vi "WPI_SonarSRF08_I2C_GetSetRefNum.vi"(8 "error in (no error)":errorcluster, 9 "menu":T1, 10 "refnum name":string, 11 "SonarSRF08_I2C_DevRef":T2={"I2CDevRef"={"DevStatus"={"status"=FALSE, "code"=0, "source"=""}, "Device Address"=0, "Handle"=0, "I2C Bus"=enum."Invalid"}} {"I2CDevRef"."Device Address" format="%.0x"}) -> (0 "error out":errorcluster, 2 "names":string[](array[string]), 3 "SonarSRF08_I2C_DevRef":T2={"I2CDevRef"={"DevStatus"={"status"=FALSE, "code"=0, "source"=""}, "Device Address"=0, "Handle"=0, "I2C Bus"=enum."Invalid"}} {"I2CDevRef"."Device Address" format="%.0x"})   [LabVIEW 2017]
doc: "Sets a reference into a registry, gets a reference from a registry, or deletes a reference from a registry. The reference is accessed by name, and can be given any unique name.\n\nThis software is licensed. Open the labview\\readme\\WPI Robotics Library Open Source License.txt file for more information."
uses:
  <vilib>/Rock Robotics/WPI/Ultrasonic/WPI_SonarSRF08_I2C_DeviceRef.ctl
  <vilib>/Rock Robotics/WPI/I2C/WPI_I2CDevRef.ctl
  <vilib>/Rock Robotics/SystemInterfaces/i2clib/i2c_bus.ctl
  <vilib>/Rock Robotics/WPI/Utilities/Refnum Registry Operation.ctl
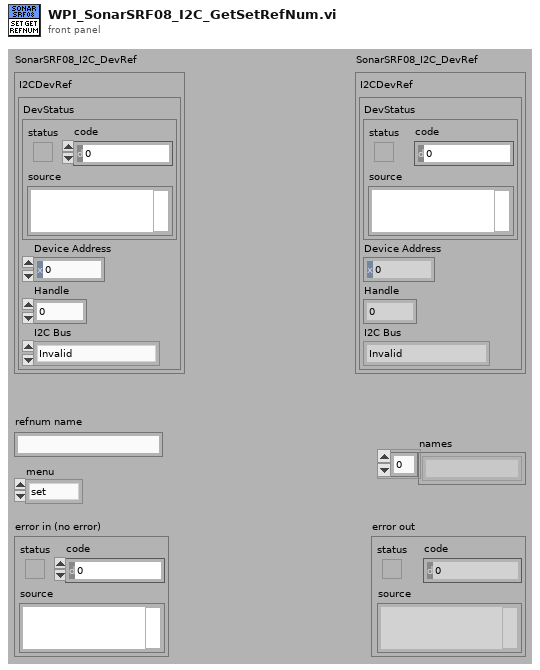
[diagram p1: front panel]
types:
  T1 = typedef "Refnum Registry Operation.ctl" = enum16{"set", "get", "delete", "get all names", "read name"}
  T2 = typedef "WPI_SonarSRF08_I2C_DeviceRef.ctl" = cluster{"I2CDevRef":T3}
  T3 = typedef "WPI_I2CDevRef.ctl" = cluster{"DevStatus":errorcluster, "Device Address":u8, "Handle":i32, "I2C Bus":T4}
  T4 = typedef "i2c_bus.ctl" = enum16{"I2C On-Board", "I2C MXP", "Invalid"}
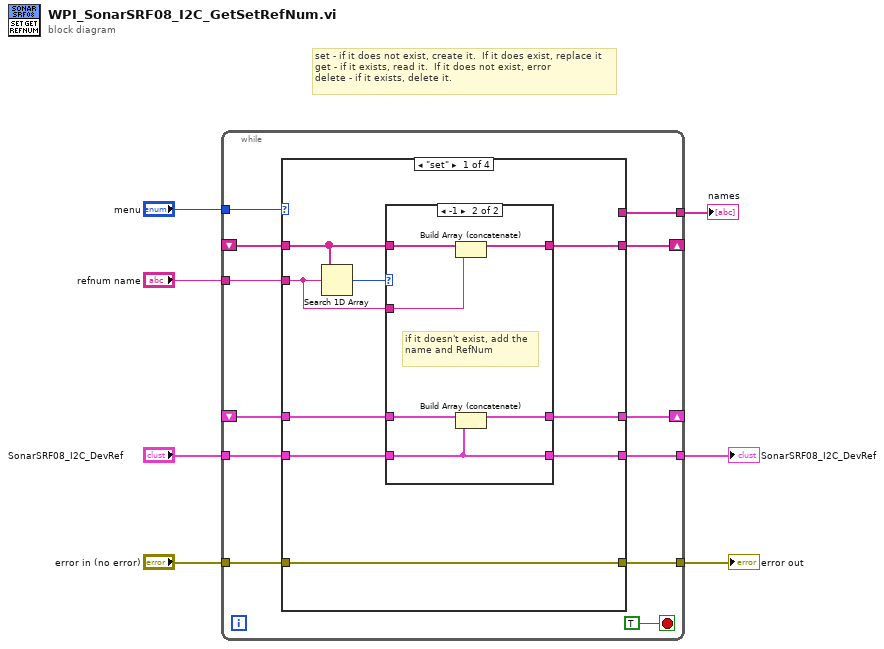
[diagram p0: block diagram]
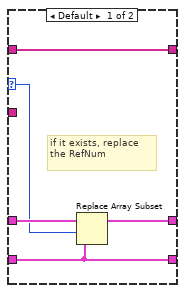
[diagram p2: hidden frame]
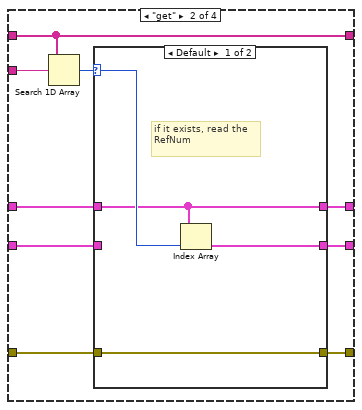
[diagram p3: hidden frame]
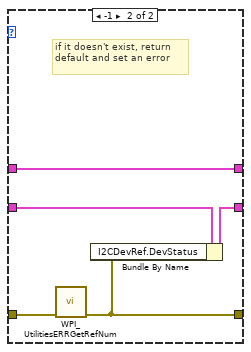
[diagram p4: hidden frame]
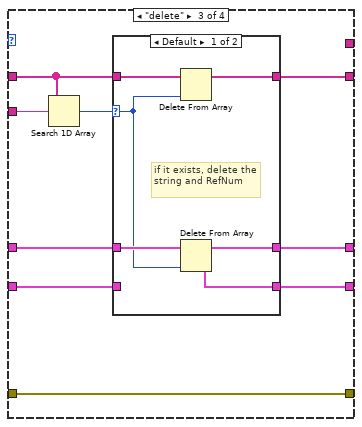
[diagram p5: hidden frame]
diagram:
  # "set - if it does not exist, create it.  If it does exist, replace it\nget - if it exists, read it.  If it does not exist, error\ndelete - if it exists, delete it."
  n1 = while {
    tunnel: "SonarSRF08_I2C_DevRef" -> [w19]
    tunnel: "refnum name" -> [w12]
    tunnel: "error in (no error)" -> [w11]
    shift-right: [w18] -> _
    shift-left: _ -> [w17]
    tunnel: [w16] -> w5
    tunnel: "menu" -> [w15]
    shift-right: [w14] -> _
    shift-left: _ -> [w13]
    tunnel: [w10] -> w3
    tunnel: [w8] -> w1
    stop <- TRUE stop-if-true
    n2 = case shown="\"set\"" w15 {
      tunnel: w19 -> [w23 w45 w61 w77]
      tunnel: [w22 w44 w60 w78] -> w18
      tunnel: w17 -> [w24 w46 w62 w78]
      tunnel: [w21 w43 w59 w77] -> w16
      tunnel: [w28 w42 w66 w79] -> w14
      tunnel: w13 -> [w27 w42 w65 w79]
      tunnel: w12 -> [w25 w47 w63 _]
      tunnel: [w20 w40 w58 w76] -> w10
      tunnel: w11 -> [w20 w41 w58 w76]
      tunnel: [_ _ _ w79] -> w8
      frame "set" {
        n3 = Search 1D Array(1D array=w27, element=w25) -> (index of element=w26:i32)  [unwired: 1 out]
        n4 = case shown="-1" w26 {
          selector: w26 -> [w31 _]
          tunnel: [w33 w39] -> w28
          tunnel: w27 -> [w33 w38]
          tunnel: w25 -> [_ w37]
          tunnel: w24 -> [w32 w36]
          tunnel: w23 -> [w29 w34]
          tunnel: [w30 w35] -> w22
          tunnel: [w29 w34] -> w21
          frame Default {
            # "if it exists, replace the RefNum"
            n5 = Replace Array Subset(array=w32, new element=w29, index=w31) -> (w30:T2[])
          }
          frame -1 {
            # "if it doesn't exist, add the name and RefNum"
            n6 = Build Array (concatenate)(w38, w37) -> (w39:string[])
            n7 = Build Array (concatenate)(w36, w34) -> (w35:T2[])
          }
        }
      }
      frame "get" {
        n8 = Search 1D Array(1D array=w42, element=w47) -> (index of element=w48:i32)  [unwired: 1 out]
        n9 = case shown="Default" w48 {
          selector: w48 -> [w52 _]
          tunnel: w46 -> [w50 w57]
          tunnel: w45 -> [_ w55]
          tunnel: [w50 w57] -> w44
          tunnel: [w51 w54] -> w43
          tunnel: w41 -> [w49 w56]
          tunnel: [w49 w53] -> w40
          frame Default {
            # "if it exists, read the RefNum"
            n10 = Index Array(array=w50, index=w52) -> (element=w51:T2)
          }
          frame -1 {
            # "if it doesn't exist, return default and set an error"
            n11 = call <vilib>:"WPI_UtilitiesERRGetRefNum.vi"("error in (no error)"=w56) -> ("ERRGetRefNum"=w53:errorcluster)  [unwired: 10 out]
            n12 = Bundle By Name(cluster=w55, "I2CDevRef.DevStatus"=w53) -> (w54:T2)
          }
        }
      }
      frame "delete" {
        n13 = Search 1D Array(1D array=w65, element=w63) -> (index of element=w64:i32)  [unwired: 1 out]
        n14 = case shown="Default" w64 {
          selector: w64 -> [w67 _]
          tunnel: [w68 w74] -> w66
          tunnel: w65 -> [w69 w74]
          tunnel: w62 -> [w72 w73]
          tunnel: w61 -> [_ w75]
          tunnel: [w71 w73] -> w60
          tunnel: [w70 w75] -> w59
          frame Default {
            # "if it exists, delete the string and RefNum"
            n15 = Delete From Array(array=w69, index=w67) -> (array with subset deleted=w68:string[])  [unwired: 1 in, 1 out]
            n16 = Delete From Array(array=w72, index=w67) -> (deleted portion=w70:T2, array with subset deleted=w71:T2[])  [unwired: 1 in]
          }
          frame -1 {
            # "if it doesn't exist, do nothing"
          }
        }
      }
      frame "get all names", Default {
      }
    }
  }
  "error out" <- w3
  "SonarSRF08_I2C_DevRef" <- w5
  "names" <- w1
